vi "Auto Move v2.vi"(8 "Current Based Move":dbl, 9 "Orientation Angle":dbl, 10 "Move Distance":dbl, 11 "Movement Angle":dbl) -> (0 "Done Moving":bool)   [LabVIEW 2017]
uses:
  Robot Global Data.vi
panel:
  out "Done Turning":bool
  in  "Turn Check Threshold":dbl=10.0
  # "Units are in Degrees"
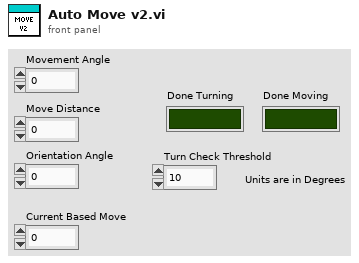
[diagram p1: front panel]
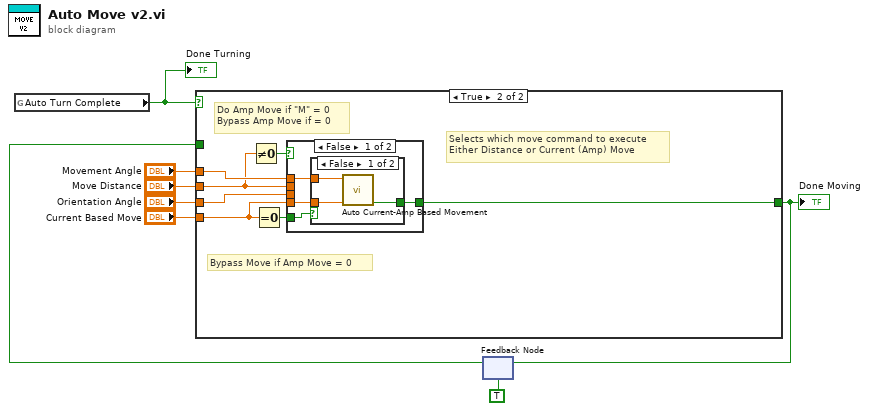
[diagram p0: block diagram]
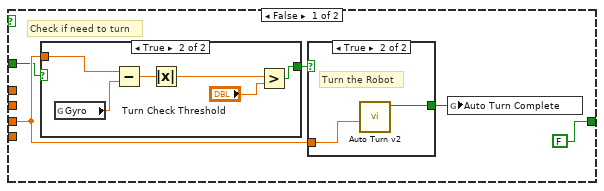
[diagram p2: hidden frame]
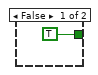
[diagram p3: hidden frame]
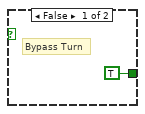
[diagram p4: hidden frame]
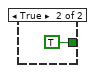
[diagram p5: hidden frame]
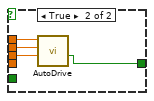
[diagram p6: hidden frame]
diagram:
  n1 = global read "Robot Global Data.vi" "Auto Turn Complete"() -> (w7:bool)
  "Done Turning" <- w7
  n2 = feedback #1(TRUE ("Done")) -> (w2:bool)
  n3 = case shown="True" w7 {
    tunnel: "Orientation Angle" -> [w12 w30]
    tunnel: "Move Distance" -> [_ w26]
    tunnel: "Movement Angle" -> [_ w29]
    tunnel: [FALSE ("Done Moving") w28] -> w3
    tunnel: "Current Based Move" -> [_ w24]
    tunnel: w2 -> [w9 _]
    frame False {
      # "Check if need to turn"
      n4 = case shown="True" w9 {
        tunnel: [TRUE w20] -> w13
        tunnel: w12 -> [_ w18]
        frame False {
        }
        frame True {
          n5 = global read "Robot Global Data.vi" "Gyro"() -> (w19:dbl)
          n6 = Subtract(x=w18, y=w19) -> (x-y=w17:dbl)
          n7 = Absolute Value(x=w17) -> (abs(x)=w16:dbl)
          n8 = Greater?(x=w16, y="Turn Check Threshold") -> (0:w20:bool)
        }
      }
      n9 = case shown="True" w13 {
        tunnel: w12 -> [_ w23]
        tunnel: [TRUE ("Done") w22] -> w11
        frame False {
          # "Bypass Turn"
        }
        frame True {
          # "Turn the Robot"
          n10 = call "Auto Turn v2.vi"("Orientation Angle"=w23) -> ("Done"=w22:bool)  [unwired: 10 in]
        }
      }
      n11 = global write "Robot Global Data.vi" "Auto Turn Complete"(w11) -> ()
    }
    frame True {
      # "Selects which move command to execute\nEither Distance or Current (Amp) Move"
      # "Do Amp Move if \"M\" = 0\nBypass Amp Move if = 0"
      # "Bypass Move if Amp Move = 0"
      n12 = Not Equal To 0?(x=w26) -> (x != 0?=w27:bool)
      n13 = Equal To 0?(x=w24) -> (x = 0?=w25:bool)
      n14 = case shown="False" w27 {
        tunnel: w30 -> [_ w42]
        tunnel: w26 -> [_ w41]
        tunnel: w29 -> [w31 w40]
        tunnel: [w34 w39] -> w28
        tunnel: w25 -> [w33 _]
        tunnel: w24 -> [w32 _]
        frame False {
          n15 = case shown="False" w33 {
            tunnel: [w37 TRUE] -> w34
            tunnel: w32 -> [w36 _]
            tunnel: w31 -> [w35 _]
            frame False {
              n16 = call "Auto Current-Amp Based Movement.vi"("Current Based Move Speed"=w36, "Movement Angle"=w35) -> ("Done Moving"=w37:bool)  [unwired: 9 in]
            }
            frame True {
            }
          }
        }
        frame True {
          n17 = call "AutoDrive.vi"("Target Robot Angle"=w42, "Distance"=w41, "Movement Angle"=w40) -> ("Done"=w39:bool)  [unwired: 8 in]
        }
      }
    }
  }
  "Done Moving" <- w3
  n18 = feedback-in #1(w3) -> ()
